vi "Update.vi"(6 "Timestamp (Now)":dbl, 8 "error in (no error)":errorcluster, 9 "Raw Value":bool, 10 "Value":bool, 11 "Channel BOOL in":refnum<class "Channel BOOL.lvclass">) -> (0 "error out":errorcluster, 3 "Channel BOOL out":refnum<class "Channel BOOL.lvclass">)   [LabVIEW 2020, in "Vecto.lvlib" / "Channel BOOL.lvclass"]
uses:
  Channel BOOL.lvclass
  Channel BOOL.lvclass/Channel BOOL.ctl
  Group BOOL/Group BOOL.lvclass
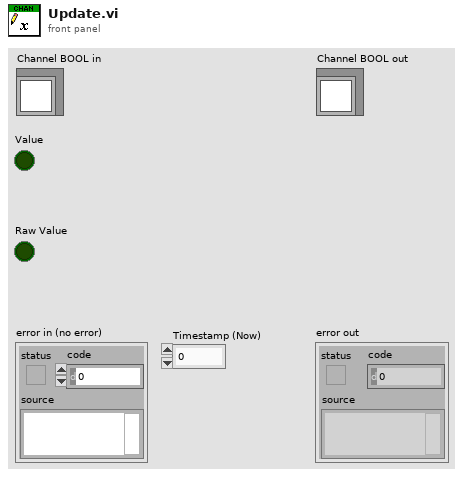
[diagram p1: front panel]
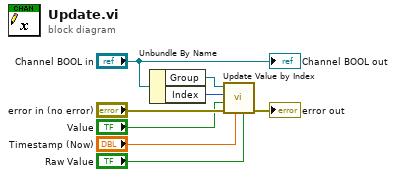
[diagram p0: block diagram]
diagram:
  n1 = Unbundle By Name("Channel BOOL in") -> ("Group"=w5:refnum<class "Group BOOL.lvclass">, "Index"=w4:i32)
  n2 = call "Update Value by Index.vi"("Raw"="Raw Value", "Timestamp (Now)"="Timestamp (Now)", "error in (no error)"="error in (no error)", "Scaled"="Value", "Index"=w4, "Group BOOL in"=w5) -> ("error out"=→"error out":errorcluster)  [unwired: 4 in, 1 out]
  "Channel BOOL out" <- "Channel BOOL in"
